vi "threhsold and centroid IMAQ.vi"(8 "error in (no error)":errorcluster, 10 "Threshold":dbl, 11 "Refnum in":T1) -> (0 "error out":errorcluster, 1 "Maximal Value":sgl, 2 "Mean Value":sgl, 3 "Refnum out":T1(plugin-control), 5 "Centroid":cluster{"X Centroid":sgl, "Y Centroid":sgl})   [LabVIEW 2013]
uses:
  IMAQ Image.ctl
  NI_Vision_Development_Module.lvlib
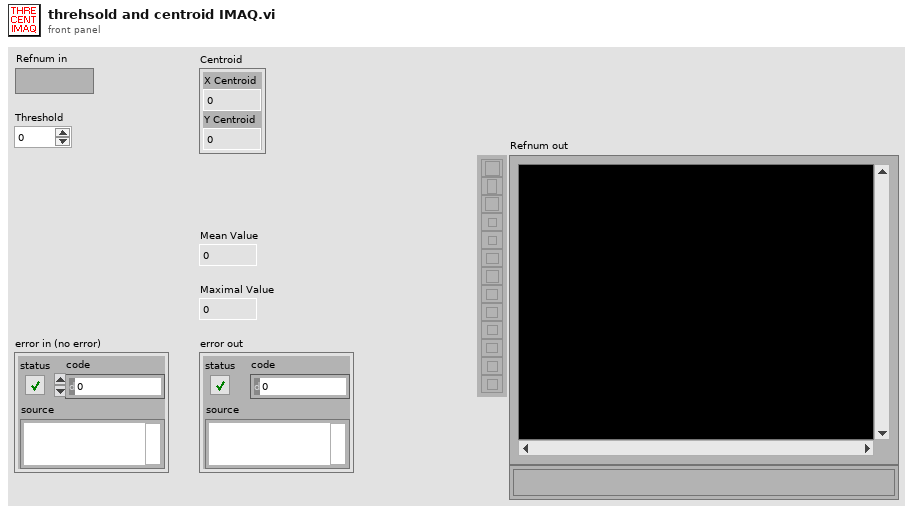
[diagram p1: front panel]
types:
  T1 = typedef "IMAQ Image.ctl" = refnum<image>
  T2 = cluster{"histogram":u32[], "Minimal Value":sgl, "Maximal Value":sgl, "Starting Value":sgl, "Interval Width":sgl, "Mean Value":sgl, "Standard  Variation":sgl, "Area (pixels)":i32}
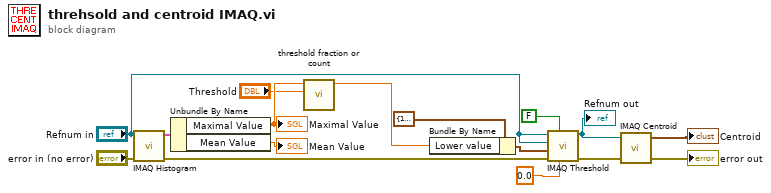
[diagram p0: block diagram]
diagram:
  n1 = call "IMAQ Histogram"("error in (no error)"="error in (no error)", "Image"="Refnum in") -> ("error out"=w7:errorcluster, "Histogram Report"=w1:T2)  [unwired: 8 in]
  n2 = Unbundle By Name(w1) -> ("Maximal Value"=w15:sgl, "Mean Value"=→"Mean Value":sgl)
  "Maximal Value" <- w15
  n3 = call "threshold fraction or count.vi"("Threshold in"="Threshold", "Maximal Value"=w15) -> ("Threshold out"=w9:dbl)  [unwired: 9 in]
  n4 = Bundle By Name(cluster=cluster{"Lower value":sgl, "Upper value":sgl} {"Lower value"=100.0, "Upper value"=9999999.0} ("Range"), "Lower value"=w9) -> (w2:cluster{"Lower value":sgl, "Upper value":sgl})
  n5 = call "IMAQ Threshold"("Replace Value"=sgl 0.0, "Keep/Replace Value (Replace)"=FALSE, "error in (no error)"=w7, "Range"=w2, "Image Dst"="Refnum in", "Image Src"="Refnum in") -> ("error out"=w8:errorcluster, "Image Dst Out"=w13:T1)  [unwired: 4 in]
  "Refnum out" <- w13
  n6 = call "IMAQ Centroid"("error in (no error)"=w8, "Image"=w13) -> ("error out"=→"error out":errorcluster, "Centroid"=→"Centroid":cluster{"X Centroid":sgl, "Y Centroid":sgl})  [unwired: 2 in]
